vi "Ballard - Arinc-429 - Add Channels.vi"(8 "error in (no error)":errorcluster, 11 "Node Ptr":u64 format="%.0x") -> (0 "error out":errorcluster)   [LabVIEW 2016, in "Ballard Arinc-429 System Explorer.lvlib"]
uses:
  Ballard Arinc-429 System Explorer.lvlib
  Shared/Controls and Global/Global.vi
  Shared/Ballard Arinc-429 Shared.lvlib
  <vilib>/NI VeriStand/Custom Device API/Custom Device API.lvlib
  <vilib>/NI Veristand/Custom Device API/Custom Device Channel Type.ctl
  <vilib>/NI Veristand/Custom Device API/Custom Device Channel.ctl
  <vilib>/NI Veristand/Custom Device API/Get Item Property (U32).vi
  Shared/Controls and Global/Start Bit.ctl
  Shared/Controls and Global/Number of Bits.ctl
  Controls/Channel Setup.ctl
panel:
  in  "Cancel":bool
  in  "OK":bool
  in  "Parameters to add":T1[](array[typedef]) {"Number of Bits" min=1 max=32}
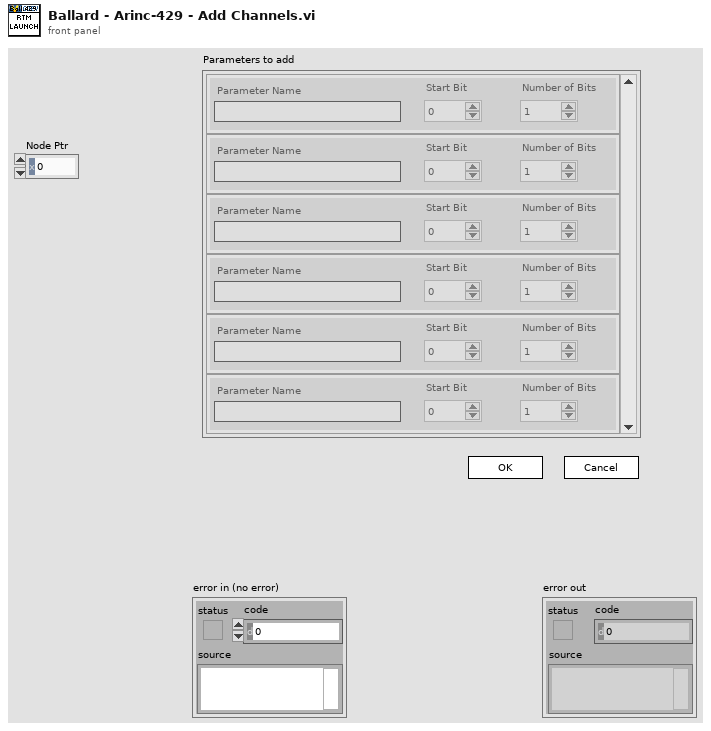
[diagram p1: front panel]
types:
  T1 = typedef "Ballard Arinc-429 System Explorer.lvlib/Channel Setup.ctl" = cluster{"Parameter Name":string, "Start Bit":T2, "Number of Bits":T3}
  T2 = typedef "Ballard Arinc-429 Shared.lvlib/Start Bit.ctl" = i32
  T3 = typedef "Ballard Arinc-429 Shared.lvlib/Number of Bits.ctl" = i32
  T4 = typedef "Custom Device API.lvlib/Custom Device Channel Type.ctl" = enum16{"Input", "Output"}
  T5 = typedef "Custom Device API.lvlib/Custom Device Channel.ctl" = cluster{"Type":T4, "Units":string, "Default Value":dbl, "Faultable":bool, "Scalable":bool}
  T6 = typedef "Custom Device API.lvlib/Custom Device Item Ref.ctl" = u64
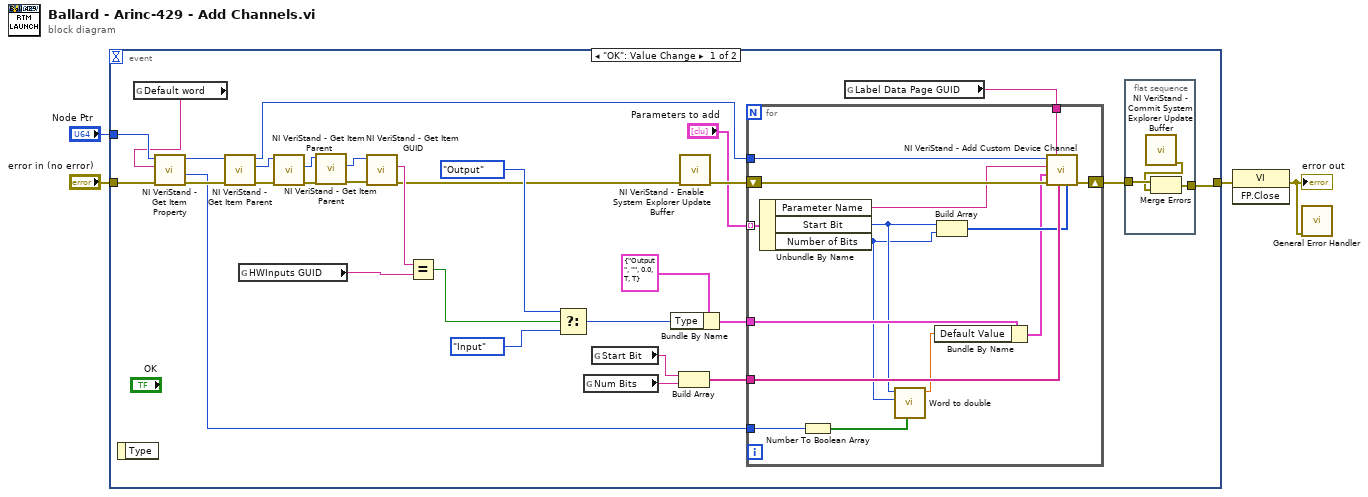
[diagram p0: block diagram]
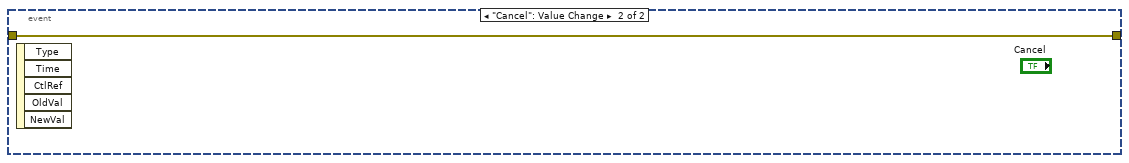
[diagram p2: hidden frame]
diagram:
  n1 = event shown="[0] \"OK\": Value Change" {
    selector: _ -> [_ _]
    dyn-events: _ -> [_ _]
    timeout: _ -> [_ _]
    tunnel: [w10 w53] -> w2
    tunnel: "error in (no error)" -> [w15 w53]
    tunnel: "Node Ptr" -> [w14 _]
    event "OK": Value Change {
      n2 = event-data() -> ()  [unwired: 1 in, 1 out]
      n3 = global read "Global.vi" "Default word"() -> (w13:string)
      n4 = call-poly <vilib>:"NI VeriStand - Get Item Property.vi"("error in (no error)"=w15, "Property Name"=w13, "Item Ref in"=w14) -> ("error out"=w17:errorcluster, "Value"=w12:u32, "Item Ref out"=w16:T6)  [unwired: 5 in, 1 out]
      n5 = call <vilib>:"NI VeriStand - Get Item Parent.vi"("error in (no error)"=w17, "Item Ref in"=w16) -> ("error out"=w31:errorcluster, "Parent Ref"=w30:T6, "Item Ref out"=w22:T6)  [unwired: 6 in, 1 out]
      n6 = global read "Global.vi" "HWInputs GUID"() -> (w24:string)
      n7 = call <vilib>:"NI VeriStand - Get Item Parent.vi"("error in (no error)"=w31, "Item Ref in"=w30) -> ("error out"=w7:errorcluster, "Parent Ref"=w6:T6)  [unwired: 6 in, 2 out]
      n8 = call <vilib>:"NI VeriStand - Get Item Parent.vi"("error in (no error)"=w7, "Item Ref in"=w6) -> ("error out"=w8:errorcluster, "Parent Ref"=w5:T6)  [unwired: 6 in, 2 out]
      n9 = call <vilib>:"NI VeriStand - Get Item GUID.vi"("error in (no error)"=w8, "Item Ref in"=w5) -> ("error out"=w9:errorcluster, "GUID"=w23:string)  [unwired: 7 in, 1 out]
      n10 = Equal?(x=w23, y=w24) -> (x = y?=w18:bool)
      n11 = Select(t=Custom_Device_Channel_Type."Output" ("Type"), s=w18, f=Custom_Device_Channel_Type."Input" ("Type")) -> (s? t:f=w27:T4)
      n12 = global read "Global.vi" "Num Bits"() -> (w33:string)
      n13 = global read "Global.vi" "Start Bit"() -> (w20:string)
      n14 = Bundle By Name(cluster=T5 {"Type"=enum."Output", "Units"="", "Default Value"=0.0, "Faultable"=TRUE, "Scalable"=TRUE} ("Channel"), "Type"=w27) -> (w29:T5)
      n15 = Build Array(w20, w33) -> (w21:string[])
      n16 = call <vilib>:"NI VeriStand - Enable System Explorer Update Buffer.vi"("error in (no error)"=w9) -> ("error out"=w34:errorcluster)  [unwired: 10 in]
      n17 = global read "Global.vi" "Label Data Page GUID"() -> (w32:string)
      n18 = for {
        shift-right: [w51] -> w11
        shift-left: w34 -> [w52]
        tunnel: w22 -> [w49]
        tunnel: w21 -> [w50]
        tunnel: w29 -> [w44]
        tunnel: w32 -> [w48]
        tunnel: "Parameters to add" -> [w47] mode=indexing
        tunnel: w12 -> [w42]
        n19 = Unbundle By Name(w47) -> ("Parameter Name"=w46:string, "Start Bit"=w40:T2, "Number of Bits"=w39:T3)
        n20 = Number To Boolean Array(number=w42) -> (Boolean array=w38:bool[])
        n21 = call "Word to double.vi"("Word"=w38, "Number of Bits"=w39, "Start Bit"=w40) -> ("Double"=w41:dbl)  [unwired: 8 in]
        n22 = Bundle By Name(cluster=w44, "Default Value"=w41) -> (w43:T5)
        n23 = Build Array(w40, w39) -> (w45:T3[])
        n24 = call <vilib>:"NI VeriStand - Add Custom Device Channel.vi"("Property Values"=w45, "Property names"=w50, "GUID (Default Channel)"=w48, "error in (no error)"=w52, "Channel"=w43, "Channel Name"=w46, "Parent Ref in"=w49) -> ("error out"=w51:errorcluster)  [unwired: 1 in, 3 out]
      }
      n25 = flat-sequence {
        tunnel: w11 -> [w37]
        tunnel: [w35] -> w10
        frame #0 {
          n26 = call <vilib>:"NI VeriStand - Commit System Explorer Update Buffer.vi"() -> ("error out"=w36:errorcluster)  [unwired: 11 in]
          n27 = Merge Errors(w37, w36) -> (w35:errorcluster)
        }
      }
    }
    event "Cancel": Value Change {
      n28 = event-data() -> ()  [unwired: 1 in, 5 out]
    }
  }
  n29 = invoke class="VI" method="FP.Close"(error in=w2) -> (error out=w1:errorcluster)  [unwired: 2 in, 2 out]
  "error out" <- w1
  n30 = call <vilib>:"General Error Handler.vi"("error in (no error)"=w1) -> ()  [unwired: 10 in, 5 out]
